vi "S4GUI.vi"(7 "Tab ObsEng":enum32{"Obs", "CCD modes", "Eng"}(tab)) -> ()   [LabVIEW 2018] (continued)
        n4313 = property on="TARGET NAME ASEL" class="Enum (strict)"() -> ("RingText.Text"=w10245:string)  [unwired: 2 in, 2 out]
        n4314 = call "Write target name.vi"("error in (no error)"=w10262, "target name"=w10245, "Optics in"=w10263) -> ("error out"=w10248:errorcluster, "Optics out"=w10249:refnum<class "Opt_Selector.lvclass">)  [unwired: 7 in]
        n4315 = Index Array(array=w10251, index="TARGET NAME ASEL") -> (element=w10250:dbl)
        n4316 = call "Write target.vi"("error in (no error)"=w10248, "target"=w10250, "Optics in"=w10249) -> ("error out"=w10247:errorcluster, "Optics out"=w10246:refnum<class "Opt_Selector.lvclass">)  [unwired: 7 in]
        n4317 = call "Write ASEL.vi"("error in (no error)"=w10247, "Opt_Selector.lvclass"=w10246, "Instrument in"=w10261) -> ("error out"=w10258:errorcluster, "Instrument out"=w10260:refnum<class "Instrument.lvclass">)  [unwired: 7 in]
        n4318 = call "Write Instrument.lvclass.vi"("error in (no error)"=w10258, "Instrument.lvclass"=w10260, "S4ACS_GUI in"=w10259) -> ("error out"=w10255:errorcluster, "S4ACS_GUI out"=w10243:refnum<class "S4GUI.lvclass">)  [unwired: 7 in]
      }
      event "WPROT_stop": Value Change {
        n4319 = event-data() -> ()  [unwired: 1 in, 4 out]
        n4320 = call "Read Instrument.lvclass.vi"("error in (no error)"=w10284, "S4ACS_GUI in"=w10285) -> ("error out"=w10282:errorcluster, "Instrument.lvclass"=w10283:refnum<class "Instrument.lvclass">, "S4ACS_GUI out"=w10269:refnum<class "S4GUI.lvclass">)  [unwired: 7 in]
        n4321 = call "Read WPROT.vi"("error in (no error)"=w10282, "Instrument in"=w10283) -> ("error out"=w10278:errorcluster, "Opt_Selector.lvclass"=w10281:refnum<class "Opt_Selector.lvclass">, "Instrument out"=w10272:refnum<class "Instrument.lvclass">)  [unwired: 7 in]
        n4322 = call-dynamic "Read State Machine.vi"("error in (no error)"=w10278, "Device in"=w10281) -> ("error out"=w10277:errorcluster, "State Machine.lvclass"=w10280:refnum<class "State Machine.lvclass">, "Device out"=w10274:refnum<class "Opt_Selector.lvclass">)  [unwired: 7 in]
        n4323 = call "Next State.vi"("error in (no error)"=w10277, "New_State"=10, "State Machine in"=w10280) -> ("error out"=w10276:errorcluster, "State Machine out"=w10275:refnum<class "State Machine.lvclass">)  [unwired: 7 in]
        n4324 = call-dynamic "Write State Machine.vi"("error in (no error)"=w10276, "State Machine.lvclass"=w10275, "Device in"=w10274) -> ("error out"=w10271:errorcluster, "Device out"=w10273:refnum<class "Opt_Selector.lvclass">)  [unwired: 7 in]
        n4325 = call "Write WPROT.vi"("error in (no error)"=w10271, "Opt_Selector.lvclass"=w10273, "Instrument in"=w10272) -> ("error out"=w10268:errorcluster, "Instrument out"=w10270:refnum<class "Instrument.lvclass">)  [unwired: 7 in]
        n4326 = call "Write Instrument.lvclass.vi"("error in (no error)"=w10268, "Instrument.lvclass"=w10270, "S4ACS_GUI in"=w10269) -> ("error out"=w10267:errorcluster, "S4ACS_GUI out"=w10266:refnum<class "S4GUI.lvclass">)  [unwired: 7 in]
      }
      event "WPROT_init": Value Change {
        n4327 = event-data() -> ()  [unwired: 1 in, 4 out]
        n4328 = call "Read Instrument.lvclass.vi"("error in (no error)"=w10304, "S4ACS_GUI in"=w10305) -> ("error out"=w10302:errorcluster, "Instrument.lvclass"=w10303:refnum<class "Instrument.lvclass">, "S4ACS_GUI out"=w10289:refnum<class "S4GUI.lvclass">)  [unwired: 7 in]
        n4329 = call "Read WPROT.vi"("error in (no error)"=w10302, "Instrument in"=w10303) -> ("error out"=w10298:errorcluster, "Opt_Selector.lvclass"=w10301:refnum<class "Opt_Selector.lvclass">, "Instrument out"=w10292:refnum<class "Instrument.lvclass">)  [unwired: 7 in]
        n4330 = call-dynamic "Read State Machine.vi"("error in (no error)"=w10298, "Device in"=w10301) -> ("error out"=w10297:errorcluster, "State Machine.lvclass"=w10300:refnum<class "State Machine.lvclass">, "Device out"=w10294:refnum<class "Opt_Selector.lvclass">)  [unwired: 7 in]
        n4331 = call "Next State.vi"("error in (no error)"=w10297, "New_State"=30, "State Machine in"=w10300) -> ("error out"=w10296:errorcluster, "State Machine out"=w10295:refnum<class "State Machine.lvclass">)  [unwired: 7 in]
        n4332 = call-dynamic "Write State Machine.vi"("error in (no error)"=w10296, "State Machine.lvclass"=w10295, "Device in"=w10294) -> ("error out"=w10291:errorcluster, "Device out"=w10293:refnum<class "Opt_Selector.lvclass">)  [unwired: 7 in]
        n4333 = call "Write WPROT.vi"("error in (no error)"=w10291, "Opt_Selector.lvclass"=w10293, "Instrument in"=w10292) -> ("error out"=w10288:errorcluster, "Instrument out"=w10290:refnum<class "Instrument.lvclass">)  [unwired: 7 in]
        n4334 = call "Write Instrument.lvclass.vi"("error in (no error)"=w10288, "Instrument.lvclass"=w10290, "S4ACS_GUI in"=w10289) -> ("error out"=w10287:errorcluster, "S4ACS_GUI out"=w10286:refnum<class "S4GUI.lvclass">)  [unwired: 7 in]
      }
      event "WPSEL_target": Value Change {
        n4335 = event-data() -> ("NewVal"=w10315:dbl)  [unwired: 1 in, 3 out]
        n4336 = call "Read Instrument.lvclass.vi"("error in (no error)"=w10319, "S4ACS_GUI in"=w10320) -> ("error out"=w10317:errorcluster, "Instrument.lvclass"=w10318:refnum<class "Instrument.lvclass">, "S4ACS_GUI out"=w10309:refnum<class "S4GUI.lvclass">)  [unwired: 7 in]
        n4337 = call "Read WPSEL.vi"("error in (no error)"=w10317, "Instrument in"=w10318) -> ("error out"=w10314:errorcluster, "Opt_Selector.lvclass"=w10316:refnum<class "Opt_Selector.lvclass">, "Instrument out"=w10312:refnum<class "Instrument.lvclass">)  [unwired: 7 in]
        n4338 = call "Write target.vi"("error in (no error)"=w10314, "target"=w10315, "Optics in"=w10316) -> ("error out"=w10311:errorcluster, "Optics out"=w10313:refnum<class "Opt_Selector.lvclass">)  [unwired: 7 in]
        n4339 = call "Write WPSEL.vi"("error in (no error)"=w10311, "Opt_Selector.lvclass"=w10313, "Instrument in"=w10312) -> ("error out"=w10308:errorcluster, "Instrument out"=w10310:refnum<class "Instrument.lvclass">)  [unwired: 7 in]
        n4340 = call "Write Instrument.lvclass.vi"("error in (no error)"=w10308, "Instrument.lvclass"=w10310, "S4ACS_GUI in"=w10309) -> ("error out"=w10307:errorcluster, "S4ACS_GUI out"=w10306:refnum<class "S4GUI.lvclass">)  [unwired: 7 in]
      }
      event "WPSEL_set": Value Change {
        n4341 = event-data() -> ()  [unwired: 1 in, 4 out]
        n4342 = call "Read Instrument.lvclass.vi"("error in (no error)"=w10339, "S4ACS_GUI in"=w10340) -> ("error out"=w10337:errorcluster, "Instrument.lvclass"=w10338:refnum<class "Instrument.lvclass">, "S4ACS_GUI out"=w10325:refnum<class "S4GUI.lvclass">)  [unwired: 7 in]
        n4343 = call "Read WPSEL.vi"("error in (no error)"=w10337, "Instrument in"=w10338) -> ("error out"=w10334:errorcluster, "Opt_Selector.lvclass"=w10336:refnum<class "Opt_Selector.lvclass">, "Instrument out"=w10328:refnum<class "Instrument.lvclass">)  [unwired: 7 in]
        n4344 = call-dynamic "Read State Machine.vi"("error in (no error)"=w10334, "Device in"=w10336) -> ("error out"=w10333:errorcluster, "State Machine.lvclass"=w10322:refnum<class "State Machine.lvclass">, "Device out"=w10330:refnum<class "Opt_Selector.lvclass">)  [unwired: 7 in]
        n4345 = call "Next State.vi"("error in (no error)"=w10333, "New_State"=1, "State Machine in"=w10322) -> ("error out"=w10332:errorcluster, "State Machine out"=w10331:refnum<class "State Machine.lvclass">)  [unwired: 7 in]
        n4346 = call-dynamic "Write State Machine.vi"("error in (no error)"=w10332, "State Machine.lvclass"=w10331, "Device in"=w10330) -> ("error out"=w10327:errorcluster, "Device out"=w10329:refnum<class "Opt_Selector.lvclass">)  [unwired: 7 in]
        n4347 = call "Write WPSEL.vi"("error in (no error)"=w10327, "Opt_Selector.lvclass"=w10329, "Instrument in"=w10328) -> ("error out"=w10324:errorcluster, "Instrument out"=w10326:refnum<class "Instrument.lvclass">)  [unwired: 7 in]
        n4348 = call "Write Instrument.lvclass.vi"("error in (no error)"=w10324, "Instrument.lvclass"=w10326, "S4ACS_GUI in"=w10325) -> ("error out"=w10323:errorcluster, "S4ACS_GUI out"=w10321:refnum<class "S4GUI.lvclass">)  [unwired: 7 in]
      }
      event "Set Waveplate": Value Change {
        # "OV20230825: Sequência de\nvalores originais."
        # "Garantir que, quando em POLARIMETRIA, pelo menos WP1 esteja selecionado."
        n4349 = event-data() -> ()  [unwired: 1 in, 4 out]
        n4350 = local read "Lambda Selector"() -> (w10444:u16)
        n4351 = property on="Calibrator Selector" class="Ring (strict)"() -> ("RingText.Text"=w10425:string)  [unwired: 2 in, 2 out]
        n4352 = call "Read Instrument.lvclass.vi"("error in (no error)"=w10424, "S4ACS_GUI in"=w10423) -> ("error out"=w10442:errorcluster, "Instrument.lvclass"=w10443:refnum<class "Instrument.lvclass">, "S4ACS_GUI out"=w10440:refnum<class "S4GUI.lvclass">)  [unwired: 7 in]
        n4353 = Build Array(0.0 ("element"), 72.0 ("element"), 144.0 ("element"), 216.0 ("element"), 288.0 ("element")) -> (w10436:dbl[])
        n4354 = local read "Calibrator Selector"() -> (w10426:u16)
        n4355 = Build Array(80.0 ("element"), 0.0 ("element"), 160.0 ("element")) -> (w10470:dbl[])
        n4356 = property on="Lambda Selector" class="Ring (strict)"() -> ("RingText.Text"=w10445:string)  [unwired: 2 in, 2 out]
        n4357 = call "Read CALW.vi"("error in (no error)"=w10442, "Instrument in"=w10443) -> ("error out"=w10434:errorcluster, "Opt_Selector.lvclass"=w10433:refnum<class "Opt_Selector.lvclass">, "Instrument out"=w10441:refnum<class "Instrument.lvclass">)  [unwired: 7 in]
        n4358 = Index Array(array=w10436, index=w10426) -> (element=w10435:dbl)
        n4359 = Index Array(array=w10470, index=w10444) -> (element=w10469:dbl)
        n4360 = case shown="\"OFF\", Default" w10425 {
          tunnel: ["OFF" w10699 "PINHOLE" "SHUTTER" w10704] -> w10343
          frame "OFF", Default {
          }
          frame "POLARIZER" {
            n4361 = disable-structure shown="Enabled" {
              disable-tunnel: ["POLARIZER" "DEPOLARIZER"] -> w10699
              frame Enabled {
              }
              frame Disabled {
                # "OV20230426: Montagem do CALW\nestá com POL e DEPOL invertidos"
              }
            }
          }
          frame "PINHOLE" {
          }
          frame "SHUTTER" {
          }
          frame "DEPOLARIZER" {
            n4362 = disable-structure shown="Enabled" {
              disable-tunnel: ["POLARIZER" "DEPOLARIZER"] -> w10704
              frame Disabled {
                # "OV20230426: Montagem do CALW\nestá com POL e DEPOL invertidos"
              }
              frame Enabled {
              }
            }
          }
        }
        n4363 = call "Write target.vi"("error in (no error)"=w10434, "target"=w10435, "Optics in"=w10433) -> ("error out"=w10431:errorcluster, "Optics out"=w10432:refnum<class "Opt_Selector.lvclass">)  [unwired: 7 in]
        n4364 = case shown="\"OFF\", Default" w10445 {
          tunnel: [w10708 "ON" "ON"] -> w10356
          tunnel: [w10707 w10709 w10712] -> w10461
          tunnel: [w10708 "L/2" "L/4"] -> w10341
          tunnel: [w10707 w10709 w10712] -> w10345
          frame "OFF", Default {
            w10708 = "OFF"
            w10707 = 0.0 ("element")
          }
          frame "Lambda/2" {
            w10709 = 30.0 ("element")
          }
          frame "Lambda/4" {
            w10712 = 30.0 ("element")
          }
        }
        n4365 = call "Write target name.vi"("error in (no error)"=w10431, "target name"=w10343, "Optics in"=w10432) -> ("error out"=w10430:errorcluster, "Optics out"=w10429:refnum<class "Opt_Selector.lvclass">)  [unwired: 7 in]
        n4366 = call "Write CALW.vi"("error in (no error)"=w10430, "Opt_Selector.lvclass"=w10429, "Instrument in"=w10441) -> ("error out"=w10427:errorcluster, "Instrument out"=w10428:refnum<class "Instrument.lvclass">)  [unwired: 7 in]
        n4367 = Equal To 0?(x=w10345) -> (x = 0?=w10346:bool)
        n4368 = call "Write Instrument.lvclass.vi"("error in (no error)"=w10427, "Instrument.lvclass"=w10428, "S4ACS_GUI in"=w10440) -> ("error out"=w10421:errorcluster, "S4ACS_GUI out"=w10422:refnum<class "S4GUI.lvclass">)  [unwired: 7 in]
        n4369 = call "Read Instrument.lvclass.vi"("error in (no error)"=w10421, "S4ACS_GUI in"=w10422) -> ("error out"=w10474:errorcluster, "Instrument.lvclass"=w10454:refnum<class "Instrument.lvclass">, "S4ACS_GUI out"=w10452:refnum<class "S4GUI.lvclass">)  [unwired: 7 in]
        n4370 = call "Read WPSEL.vi"("error in (no error)"=w10474, "Instrument in"=w10454) -> ("error out"=w10460:errorcluster, "Opt_Selector.lvclass"=w10459:refnum<class "Opt_Selector.lvclass">, "Instrument out"=w10453:refnum<class "Instrument.lvclass">)  [unwired: 7 in]
        n4371 = call "Write target.vi"("error in (no error)"=w10460, "target"=w10469, "Optics in"=w10459) -> ("error out"=w10457:errorcluster, "Optics out"=w10458:refnum<class "Opt_Selector.lvclass">)  [unwired: 7 in]
        n4372 = call "Write target name.vi"("error in (no error)"=w10457, "target name"=w10341, "Optics in"=w10458) -> ("error out"=w10456:errorcluster, "Optics out"=w10455:refnum<class "Opt_Selector.lvclass">)  [unwired: 7 in]
        n4373 = call "Write WPSEL.vi"("error in (no error)"=w10456, "Opt_Selector.lvclass"=w10455, "Instrument in"=w10453) -> ("error out"=w10449:errorcluster, "Instrument out"=w10448:refnum<class "Instrument.lvclass">)  [unwired: 7 in]
        n4374 = call "Read ASEL.vi"("error in (no error)"=w10449, "Instrument in"=w10448) -> ("error out"=w10466:errorcluster, "Opt_Selector.lvclass"=w10464:refnum<class "Opt_Selector.lvclass">, "Instrument out"=w10451:refnum<class "Instrument.lvclass">)  [unwired: 7 in]
        n4375 = call "Write target name.vi"("error in (no error)"=w10466, "target name"=w10356, "Optics in"=w10464) -> ("error out"=w10467:errorcluster, "Optics out"=w10463:refnum<class "Opt_Selector.lvclass">)  [unwired: 7 in]
        n4376 = Select(t="OFF", s=w10346, f=w10343) -> (s? t:f=w10344:string)
        n4377 = call "Write target.vi"("error in (no error)"=w10467, "target"=w10461, "Optics in"=w10463) -> ("error out"=w10468:errorcluster, "Optics out"=w10462:refnum<class "Opt_Selector.lvclass">)  [unwired: 7 in]
        n4378 = call "Write ASEL.vi"("error in (no error)"=w10468, "Opt_Selector.lvclass"=w10462, "Instrument in"=w10451) -> ("error out"=w10465:errorcluster, "Instrument out"=w10450:refnum<class "Instrument.lvclass">)  [unwired: 7 in]
        n4379 = call "Write Instrument.lvclass.vi"("error in (no error)"=w10465, "Instrument.lvclass"=w10450, "S4ACS_GUI in"=w10452) -> ("error out"=w10446:errorcluster, "S4ACS_GUI out"=w10447:refnum<class "S4GUI.lvclass">)  [unwired: 7 in]
        n4380 = call "Read Instrument.lvclass.vi"("error in (no error)"=w10446, "S4ACS_GUI in"=w10447) -> ("error out"=w10515:errorcluster, "Instrument.lvclass"=w10516:refnum<class "Instrument.lvclass">, "S4ACS_GUI out"=w10362:refnum<class "S4GUI.lvclass">)  [unwired: 7 in]
        n4381 = call "Read WPSEL.vi"("error in (no error)"=w10515, "Instrument in"=w10516) -> ("error out"=w10512:errorcluster, "Opt_Selector.lvclass"=w10514:refnum<class "Opt_Selector.lvclass">, "Instrument out"=w10506:refnum<class "Instrument.lvclass">)  [unwired: 7 in]
        n4382 = call-dynamic "Read State Machine.vi"("error in (no error)"=w10512, "Device in"=w10514) -> ("error out"=w10511:errorcluster, "State Machine.lvclass"=w10504:refnum<class "State Machine.lvclass">, "Device out"=w10508:refnum<class "Opt_Selector.lvclass">)  [unwired: 7 in]
        n4383 = call "Next State.vi"("error in (no error)"=w10511, "New_State"=1, "State Machine in"=w10504) -> ("error out"=w10510:errorcluster, "State Machine out"=w10509:refnum<class "State Machine.lvclass">)  [unwired: 7 in]
        n4384 = call-dynamic "Write State Machine.vi"("error in (no error)"=w10510, "State Machine.lvclass"=w10509, "Device in"=w10508) -> ("error out"=w10505:errorcluster, "Device out"=w10507:refnum<class "Opt_Selector.lvclass">)  [unwired: 7 in]
        n4385 = call "Write WPSEL.vi"("error in (no error)"=w10505, "Opt_Selector.lvclass"=w10507, "Instrument in"=w10506) -> ("error out"=w10496:errorcluster, "Instrument out"=w10495:refnum<class "Instrument.lvclass">)  [unwired: 7 in]
        n4386 = call "Read ASEL.vi"("error in (no error)"=w10496, "Instrument in"=w10495) -> ("error out"=w10502:errorcluster, "Opt_Selector.lvclass"=w10493:refnum<class "Opt_Selector.lvclass">, "Instrument out"=w10494:refnum<class "Instrument.lvclass">)  [unwired: 7 in]
        n4387 = call-dynamic "Read State Machine.vi"("error in (no error)"=w10502, "Device in"=w10493) -> ("error out"=w10501:errorcluster, "State Machine.lvclass"=w10497:refnum<class "State Machine.lvclass">, "Device out"=w10492:refnum<class "Opt_Selector.lvclass">)  [unwired: 7 in]
        n4388 = call "Next State.vi"("error in (no error)"=w10501, "New_State"=1, "State Machine in"=w10497) -> ("error out"=w10500:errorcluster, "State Machine out"=w10499:refnum<class "State Machine.lvclass">)  [unwired: 7 in]
        n4389 = call-dynamic "Write State Machine.vi"("error in (no error)"=w10500, "State Machine.lvclass"=w10499, "Device in"=w10492) -> ("error out"=w10498:errorcluster, "Device out"=w10491:refnum<class "Opt_Selector.lvclass">)  [unwired: 7 in]
        n4390 = Concatenate Strings("SET WAVEPLATE:  WPSEL=" ("string"), w10341, " CALW=" ("string"), w10344) -> (w10354:string)
        n4391 = call "Write ASEL.vi"("error in (no error)"=w10498, "Opt_Selector.lvclass"=w10491, "Instrument in"=w10494) -> ("error out"=w10478:errorcluster, "Instrument out"=w10480:refnum<class "Instrument.lvclass">)  [unwired: 7 in]
        n4392 = call "Read CALW.vi"("error in (no error)"=w10478, "Instrument in"=w10480) -> ("error out"=w10488:errorcluster, "Opt_Selector.lvclass"=w10490:refnum<class "Opt_Selector.lvclass">, "Instrument out"=w10479:refnum<class "Instrument.lvclass">)  [unwired: 7 in]
        n4393 = call-dynamic "Read State Machine.vi"("error in (no error)"=w10488, "Device in"=w10490) -> ("error out"=w10487:errorcluster, "State Machine.lvclass"=w10481:refnum<class "State Machine.lvclass">, "Device out"=w10484:refnum<class "Opt_Selector.lvclass">)  [unwired: 7 in]
        n4394 = call "Next State.vi"("error in (no error)"=w10487, "New_State"=1, "State Machine in"=w10481) -> ("error out"=w10486:errorcluster, "State Machine out"=w10485:refnum<class "State Machine.lvclass">)  [unwired: 7 in]
        n4395 = call-dynamic "Write State Machine.vi"("error in (no error)"=w10486, "State Machine.lvclass"=w10485, "Device in"=w10484) -> ("error out"=w10482:errorcluster, "Device out"=w10483:refnum<class "Opt_Selector.lvclass">)  [unwired: 7 in]
        n4396 = property on="Lambda Selector" class="Ring (strict)"() -> ("RingText.Text"=w10477:string)  [unwired: 2 in, 2 out]
        n4397 = call "Write CALW.vi"("error in (no error)"=w10482, "Opt_Selector.lvclass"=w10483, "Instrument in"=w10479) -> ("error out"=w10361:errorcluster, "Instrument out"=w10476:refnum<class "Instrument.lvclass">)  [unwired: 7 in]
        n4398 = call-dynamic "Read mode EXPOSE.vi"("error in (no error)"=w10361, "S4GUI in"=w10362) -> ("error out"=w10360:errorcluster, "mode EXPOSE"=w10358:bool, "S4GUI out"=w10359:refnum<class "S4GUI.lvclass">)  [unwired: 7 in]
        n4399 = call-dynamic "Read sync.vi"("error in (no error)"=w10360, "S4ACS_GUI in"=w10359) -> ("error out"=w10378:errorcluster, "sync"=w10377:bool, "S4ACS_GUI out"=w10379:refnum<class "S4GUI.lvclass">)  [unwired: 7 in]
        n4400 = case shown="\"OFF\"" w10477 {
          selector: w10477 -> [w10724 _]
          tunnel: w10476 -> [w10728 w10746]
          tunnel: [w10727 w10746] -> w10475
          tunnel: [w10720 w10745] -> w10395
          tunnel: w10378 -> [w10726 w10745]
          tunnel: [w10717 w10741] -> w10390
          tunnel: w10377 -> [w10716 _]
          tunnel: w10358 -> [w10715 w10744]
          frame "OFF" {
            w10718 = u16 0 items=["OFF", "POLARIZER", "PINHOLE", "SHUTTER", "DEPOLARIZER"] ("Calibrator Selector 2")
            n4401 = call "Read CALW.vi"("error in (no error)"=w10726, "Instrument in"=w10728) -> ("error out"=w10731:errorcluster, "Opt_Selector.lvclass"=w10733:refnum<class "Opt_Selector.lvclass">, "Instrument out"=w10732:refnum<class "Instrument.lvclass">)  [unwired: 7 in]
            n4402 = call "Write target.vi"("error in (no error)"=w10731, "target"=0.0, "Optics in"=w10733) -> ("error out"=w10730:errorcluster, "Optics out"=w10734:refnum<class "Opt_Selector.lvclass">)  [unwired: 7 in]
            n4403 = call "Write target name.vi"("error in (no error)"=w10730, "target name"=w10724, "Optics in"=w10734) -> ("error out"=w10729:errorcluster, "Optics out"=w10735:refnum<class "Opt_Selector.lvclass">)  [unwired: 7 in]
            n4404 = call "Write CALW.vi"("error in (no error)"=w10729, "Opt_Selector.lvclass"=w10735, "Instrument in"=w10732) -> ("error out"=w10719:errorcluster, "Instrument out"=w10727:refnum<class "Instrument.lvclass">)  [unwired: 7 in]
            n4405 = property on="Calibrator Selector" class="Ring (strict)"(error in=w10719, "Value"=w10718, "DisabledEnum"=T12."Disabled and Grayed Out" ("Disabled")) -> (error out=w10721:errorcluster)  [unwired: 1 in, 1 out]
            n4406 = property on="Calibrator Selector" class="Ring (strict)"(error in=w10721, "RingText.Text"="OFF" ("Ring Text.Text")) -> (error out=w10720:errorcluster)  [unwired: 1 in, 1 out]
            n4407 = case shown="True" w10716 {
              tunnel: [u8 0 ("SHUTTER_MODE") w10738] -> w10717
              tunnel: w10715 -> [_ w10737]
              frame False {
                # "Fotom. & Async"
                # "Internal"
              }
              frame True {
                # "Ext. Start"
                # "Internal"
                # "Fotom. Sync. SEM exp mode"
                # "Fotom. Sync. COM exp mode"
                n4408 = Select(t=u8 0, s=w10737, f=u8 6 ("SHUTTER_MODE")) -> (s? t:f=w10738:u8)
              }
            }
          }
          frame Default {
            # "Polar. COM exp mode"
            # "Internal"
            # "Polar. SEM exp mode"
            # "Ext. Start"
            n4409 = Select(t=u8 0, s=w10744, f=u8 6 ("SHUTTER_MODE")) -> (s? t:f=w10741:u8)
          }
        }
        n4410 = call "Write Instrument.lvclass.vi"("error in (no error)"=w10395, "Instrument.lvclass"=w10475, "S4ACS_GUI in"=w10379) -> ("error out"=w10394:errorcluster, "S4ACS_GUI out"=w10383:refnum<class "S4GUI.lvclass">)  [unwired: 7 in]
        n4411 = call-dynamic "Read AcquisitionC.vi"("error in (no error)"=w10394, "S4ACS_GUI in"=w10383) -> ("error out"=w10405:errorcluster, "Acquisition.lvclass"=w10404:refnum<class "Acquisition.lvclass">)  [unwired: 7 in, 1 out]
        n4412 = call-dynamic "Read AcquisitionA.vi"("error in (no error)"=w10394, "S4ACS_GUI in"=w10383) -> ("error out"=w10408:errorcluster, "Acquisition.lvclass"=w10409:refnum<class "Acquisition.lvclass">)  [unwired: 7 in, 1 out]
        n4413 = call "Read AcquisitionB.vi"("error in (no error)"=w10394, "S4ACS_GUI in"=w10383) -> ("error out"=w10406:errorcluster, "Acquisition.lvclass"=w10407:refnum<class "Acquisition.lvclass">)  [unwired: 7 in, 1 out]
        n4414 = call-dynamic "Read AcquisitionD.vi"("error in (no error)"=w10394, "S4ACS_GUI in"=w10383) -> ("error out"=w10402:errorcluster, "Acquisition.lvclass"=w10403:refnum<class "Acquisition.lvclass">)  [unwired: 7 in, 1 out]
        n4415 = call "Read connection.vi"("error in (no error)"=w10405, "Server in"=w10404) -> ("error out"=w10411:errorcluster, "connection"=w10410:bool, "Server out"=w10412:refnum<class "Acquisition.lvclass">)  [unwired: 7 in]
        n4416 = call "Read connection.vi"("error in (no error)"=w10406, "Server in"=w10407) -> ("error out"=w10414:errorcluster, "connection"=w10413:bool, "Server out"=w10415:refnum<class "Acquisition.lvclass">)  [unwired: 7 in]
        n4417 = call "Read connection.vi"("error in (no error)"=w10402, "Server in"=w10403) -> ("error out"=w10391:errorcluster, "connection"=w10392:bool, "Server out"=w10393:refnum<class "Acquisition.lvclass">)  [unwired: 7 in]
        n4418 = call "Read connection.vi"("error in (no error)"=w10408, "Server in"=w10409) -> ("error out"=w10417:errorcluster, "connection"=w10416:bool, "Server out"=w10418:refnum<class "Acquisition.lvclass">)  [unwired: 7 in]
        n4419 = case shown="True" w10410 {
          tunnel: w10412 -> [w10582 w10587]
          tunnel: w10411 -> [w10581 w10586]
          tunnel: [w10582 w10585] -> w10397
          tunnel: [w10581 w10584] -> w10396
          tunnel: w10390 -> [_ w10583]
          frame False {
          }
          frame True {
            # "nome do arquivo .cfg"
            # "seção no arquivo .cfg"
            n4420 = call-dynamic "Read Channel.vi"("error in (no error)"=w10586, "Acquisition in"=w10587) -> ("error out"=w10591:errorcluster, "Channel.lvclass"=w10590:refnum<class "Channel.lvclass">, "Acquisition out"=w10589:refnum<class "Acquisition.lvclass">)  [unwired: 7 in]
            n4421 = call-dynamic "Read Interface.vi"("error in (no error)"=w10591, "Channel in"=w10590) -> ("error out"=w10598:errorcluster, "Interface.lvclass"=w10599:refnum<class "Interface.lvclass">, "Channel out"=w10588:refnum<class "Channel.lvclass">)  [unwired: 7 in]
            n4422 = call-dynamic "Get CCD_Config.vi"("error in (no error)"=w10598, "Interface in"=w10599) -> ("error out"=w10596:errorcluster, "output cluster"=w10595:T30, "Interface out"=w10600:refnum<class "Interface.lvclass">)  [unwired: 7 in]
            n4423 = Bundle By Name(cluster=w10595, "TRIGGER_MODE"=w10583) -> (w10597:T30)
            n4424 = call-dynamic "Set CCD_Config.vi"("error in (no error)"=w10596, "input cluster"=w10597, "Interface in"=w10600) -> ("error out"=w10594:errorcluster, "Interface out"=w10601:refnum<class "Interface.lvclass">)  [unwired: 7 in]
            n4425 = Flatten To String(anything=w10597, error in (no error)=w10594) -> (data string=w10592:string, error out=w10593:errorcluster)  [unwired: 2 in, 1 out]
            n4426 = call "Write flatted cluster.vi"("error in (no error)"=w10593, "flatted cluster"=w10592, "Interface in"=w10601) -> ("error out"=w10603:errorcluster, "Interface out"=w10602:refnum<class "Interface.lvclass">)  [unwired: 7 in]
            n4427 = call-dynamic "Write Interface.vi"("error in (no error)"=w10603, "Interface.lvclass"=w10602, "Channel in"=w10588) -> ("error out"=w10609:errorcluster, "Channel out"=w10610:refnum<class "Channel.lvclass">)  [unwired: 7 in]
            n4428 = call "Write section_name.vi"("error in (no error)"=w10609, "section_name"="CCD_ACS3", "Channel in"=w10610) -> ("error out"=w10607:errorcluster, "Channel out"=w10613:refnum<class "Channel.lvclass">)  [unwired: 7 in]
            n4429 = call-dynamic "save config.vi"("error in (no error)"=w10607, "file config"="lastsaved.cfg", "Channel in"=w10613) -> ("error out"=w10608:errorcluster, "Channel out"=w10614:refnum<class "Channel.lvclass">)  [unwired: 7 in]
            n4430 = call-dynamic "Read State Machine.vi"("error in (no error)"=w10608, "Device in"=w10614) -> ("error out"=w10604:errorcluster, "State Machine.lvclass"=w10616:refnum<class "State Machine.lvclass">, "Device out"=w10615:refnum<class "Channel.lvclass">)  [unwired: 7 in]
            n4431 = call-dynamic "Write State.vi"("error in (no error)"=w10604, "State"=60, "State Machine in"=w10616) -> ("error out"=w10605:errorcluster, "State Machine out"=w10617:refnum<class "State Machine.lvclass">)  [unwired: 7 in]
            n4432 = call-dynamic "Write State Machine.vi"("error in (no error)"=w10605, "State Machine.lvclass"=w10617, "Device in"=w10615) -> ("error out"=w10619:errorcluster, "Device out"=w10618:refnum<class "Channel.lvclass">)  [unwired: 7 in]
            n4433 = call-dynamic "Write Channel.vi"("error in (no error)"=w10619, "Channel.lvclass"=w10618, "Acquisition in"=w10589) -> ("error out"=w10584:errorcluster, "Acquisition out"=w10585:refnum<class "Acquisition.lvclass">)  [unwired: 7 in]
          }
        }
        n4434 = case shown="True" w10392 {
          tunnel: w10393 -> [w10543 w10548]
          tunnel: w10391 -> [w10542 w10547]
          tunnel: w10390 -> [_ w10546]
          tunnel: [w10543 w10545] -> w10389
          tunnel: [w10542 w10544] -> w10388
          frame False {
          }
          frame True {
            # "nome do arquivo .cfg"
            # "seção no arquivo .cfg"
            n4435 = call-dynamic "Read Channel.vi"("error in (no error)"=w10547, "Acquisition in"=w10548) -> ("error out"=w10577:errorcluster, "Channel.lvclass"=w10578:refnum<class "Channel.lvclass">, "Acquisition out"=w10579:refnum<class "Acquisition.lvclass">)  [unwired: 7 in]
            n4436 = call-dynamic "Read Interface.vi"("error in (no error)"=w10577, "Channel in"=w10578) -> ("error out"=w10570:errorcluster, "Interface.lvclass"=w10569:refnum<class "Interface.lvclass">, "Channel out"=w10580:refnum<class "Channel.lvclass">)  [unwired: 7 in]
            n4437 = call-dynamic "Get CCD_Config.vi"("error in (no error)"=w10570, "Interface in"=w10569) -> ("error out"=w10572:errorcluster, "output cluster"=w10573:T30, "Interface out"=w10568:refnum<class "Interface.lvclass">)  [unwired: 7 in]
            n4438 = Bundle By Name(cluster=w10573, "TRIGGER_MODE"=w10546) -> (w10571:T30)
            n4439 = call-dynamic "Set CCD_Config.vi"("error in (no error)"=w10572, "input cluster"=w10571, "Interface in"=w10568) -> ("error out"=w10574:errorcluster, "Interface out"=w10567:refnum<class "Interface.lvclass">)  [unwired: 7 in]
            n4440 = Flatten To String(anything=w10571, error in (no error)=w10574) -> (data string=w10576:string, error out=w10575:errorcluster)  [unwired: 2 in, 1 out]
            n4441 = call "Write flatted cluster.vi"("error in (no error)"=w10575, "flatted cluster"=w10576, "Interface in"=w10567) -> ("error out"=w10565:errorcluster, "Interface out"=w10566:refnum<class "Interface.lvclass">)  [unwired: 7 in]
            n4442 = call-dynamic "Write Interface.vi"("error in (no error)"=w10565, "Interface.lvclass"=w10566, "Channel in"=w10580) -> ("error out"=w10559:errorcluster, "Channel out"=w10558:refnum<class "Channel.lvclass">)  [unwired: 7 in]
            n4443 = call "Write section_name.vi"("error in (no error)"=w10559, "section_name"="CCD_ACS4", "Channel in"=w10558) -> ("error out"=w10561:errorcluster, "Channel out"=w10555:refnum<class "Channel.lvclass">)  [unwired: 7 in]
            n4444 = call-dynamic "save config.vi"("error in (no error)"=w10561, "file config"="lastsaved.cfg", "Channel in"=w10555) -> ("error out"=w10560:errorcluster, "Channel out"=w10554:refnum<class "Channel.lvclass">)  [unwired: 7 in]
            n4445 = call-dynamic "Read State Machine.vi"("error in (no error)"=w10560, "Device in"=w10554) -> ("error out"=w10564:errorcluster, "State Machine.lvclass"=w10552:refnum<class "State Machine.lvclass">, "Device out"=w10553:refnum<class "Channel.lvclass">)  [unwired: 7 in]
            n4446 = call-dynamic "Write State.vi"("error in (no error)"=w10564, "State"=60, "State Machine in"=w10552) -> ("error out"=w10563:errorcluster, "State Machine out"=w10551:refnum<class "State Machine.lvclass">)  [unwired: 7 in]
            n4447 = call-dynamic "Write State Machine.vi"("error in (no error)"=w10563, "State Machine.lvclass"=w10551, "Device in"=w10553) -> ("error out"=w10549:errorcluster, "Device out"=w10550:refnum<class "Channel.lvclass">)  [unwired: 7 in]
            n4448 = call-dynamic "Write Channel.vi"("error in (no error)"=w10549, "Channel.lvclass"=w10550, "Acquisition in"=w10579) -> ("error out"=w10544:errorcluster, "Acquisition out"=w10545:refnum<class "Acquisition.lvclass">)  [unwired: 7 in]
          }
        }
        n4449 = case shown="True" w10413 {
          tunnel: w10415 -> [w10621 w10626]
          tunnel: w10414 -> [w10620 w10625]
          tunnel: [w10621 w10624] -> w10399
          tunnel: [w10620 w10623] -> w10398
          tunnel: w10390 -> [_ w10622]
          frame False {
          }
          frame True {
            # "nome do arquivo .cfg"
            # "seção no arquivo .cfg"
            n4450 = call-dynamic "Read Channel.vi"("error in (no error)"=w10625, "Acquisition in"=w10626) -> ("error out"=w10630:errorcluster, "Channel.lvclass"=w10629:refnum<class "Channel.lvclass">, "Acquisition out"=w10628:refnum<class "Acquisition.lvclass">)  [unwired: 7 in]
            n4451 = call-dynamic "Read Interface.vi"("error in (no error)"=w10630, "Channel in"=w10629) -> ("error out"=w10637:errorcluster, "Interface.lvclass"=w10638:refnum<class "Interface.lvclass">, "Channel out"=w10627:refnum<class "Channel.lvclass">)  [unwired: 7 in]
            n4452 = call-dynamic "Get CCD_Config.vi"("error in (no error)"=w10637, "Interface in"=w10638) -> ("error out"=w10635:errorcluster, "output cluster"=w10634:T30, "Interface out"=w10639:refnum<class "Interface.lvclass">)  [unwired: 7 in]
            n4453 = Bundle By Name(cluster=w10634, "TRIGGER_MODE"=w10622) -> (w10636:T30)
            n4454 = call-dynamic "Set CCD_Config.vi"("error in (no error)"=w10635, "input cluster"=w10636, "Interface in"=w10639) -> ("error out"=w10633:errorcluster, "Interface out"=w10640:refnum<class "Interface.lvclass">)  [unwired: 7 in]
            n4455 = Flatten To String(anything=w10636, error in (no error)=w10633) -> (data string=w10631:string, error out=w10632:errorcluster)  [unwired: 2 in, 1 out]
            n4456 = call "Write flatted cluster.vi"("error in (no error)"=w10632, "flatted cluster"=w10631, "Interface in"=w10640) -> ("error out"=w10642:errorcluster, "Interface out"=w10641:refnum<class "Interface.lvclass">)  [unwired: 7 in]
            n4457 = call-dynamic "Write Interface.vi"("error in (no error)"=w10642, "Interface.lvclass"=w10641, "Channel in"=w10627) -> ("error out"=w10648:errorcluster, "Channel out"=w10649:refnum<class "Channel.lvclass">)  [unwired: 7 in]
            n4458 = call "Write section_name.vi"("error in (no error)"=w10648, "section_name"="CCD_ACS2", "Channel in"=w10649) -> ("error out"=w10646:errorcluster, "Channel out"=w10652:refnum<class "Channel.lvclass">)  [unwired: 7 in]
            n4459 = call-dynamic "save config.vi"("error in (no error)"=w10646, "file config"="lastsaved.cfg", "Channel in"=w10652) -> ("error out"=w10647:errorcluster, "Channel out"=w10653:refnum<class "Channel.lvclass">)  [unwired: 7 in]
            n4460 = call-dynamic "Read State Machine.vi"("error in (no error)"=w10647, "Device in"=w10653) -> ("error out"=w10643:errorcluster, "State Machine.lvclass"=w10655:refnum<class "State Machine.lvclass">, "Device out"=w10654:refnum<class "Channel.lvclass">)  [unwired: 7 in]
            n4461 = call-dynamic "Write State.vi"("error in (no error)"=w10643, "State"=60, "State Machine in"=w10655) -> ("error out"=w10644:errorcluster, "State Machine out"=w10656:refnum<class "State Machine.lvclass">)  [unwired: 7 in]
            n4462 = call-dynamic "Write State Machine.vi"("error in (no error)"=w10644, "State Machine.lvclass"=w10656, "Device in"=w10654) -> ("error out"=w10658:errorcluster, "Device out"=w10657:refnum<class "Channel.lvclass">)  [unwired: 7 in]
            n4463 = call-dynamic "Write Channel.vi"("error in (no error)"=w10658, "Channel.lvclass"=w10657, "Acquisition in"=w10628) -> ("error out"=w10623:errorcluster, "Acquisition out"=w10624:refnum<class "Acquisition.lvclass">)  [unwired: 7 in]
          }
        }
        n4464 = case shown="True" w10416 {
          tunnel: [w10659 w10693] -> w10400
          tunnel: [w10660 w10692] -> w10401
          tunnel: w10418 -> [w10660 w10663]
          tunnel: w10417 -> [w10659 w10662]
          tunnel: w10390 -> [_ w10661]
          frame False {
          }
          frame True {
            # "nome do arquivo .cfg"
            # "seção no arquivo .cfg"
            n4465 = call-dynamic "Read Channel.vi"("error in (no error)"=w10662, "Acquisition in"=w10663) -> ("error out"=w10694:errorcluster, "Channel.lvclass"=w10695:refnum<class "Channel.lvclass">, "Acquisition out"=w10696:refnum<class "Acquisition.lvclass">)  [unwired: 7 in]
            n4466 = call-dynamic "Read Interface.vi"("error in (no error)"=w10694, "Channel in"=w10695) -> ("error out"=w10685:errorcluster, "Interface.lvclass"=w10684:refnum<class "Interface.lvclass">, "Channel out"=w10697:refnum<class "Channel.lvclass">)  [unwired: 7 in]
            n4467 = call-dynamic "Get CCD_Config.vi"("error in (no error)"=w10685, "Interface in"=w10684) -> ("error out"=w10687:errorcluster, "output cluster"=w10688:T30, "Interface out"=w10683:refnum<class "Interface.lvclass">)  [unwired: 7 in]
            n4468 = Bundle By Name(cluster=w10688, "TRIGGER_MODE"=w10661) -> (w10686:T30)
            n4469 = call-dynamic "Set CCD_Config.vi"("error in (no error)"=w10687, "input cluster"=w10686, "Interface in"=w10683) -> ("error out"=w10689:errorcluster, "Interface out"=w10682:refnum<class "Interface.lvclass">)  [unwired: 7 in]
            n4470 = Flatten To String(anything=w10686, error in (no error)=w10689) -> (data string=w10691:string, error out=w10690:errorcluster)  [unwired: 2 in, 1 out]
            n4471 = call "Write flatted cluster.vi"("error in (no error)"=w10690, "flatted cluster"=w10691, "Interface in"=w10682) -> ("error out"=w10680:errorcluster, "Interface out"=w10681:refnum<class "Interface.lvclass">)  [unwired: 7 in]
            n4472 = call-dynamic "Write Interface.vi"("error in (no error)"=w10680, "Interface.lvclass"=w10681, "Channel in"=w10697) -> ("error out"=w10675:errorcluster, "Channel out"=w10674:refnum<class "Channel.lvclass">)  [unwired: 7 in]
            n4473 = call "Write section_name.vi"("error in (no error)"=w10675, "section_name"="CCD_ACS1", "Channel in"=w10674) -> ("error out"=w10676:errorcluster, "Channel out"=w10671:refnum<class "Channel.lvclass">)  [unwired: 7 in]
            n4474 = call-dynamic "save config.vi"("error in (no error)"=w10676, "file config"="lastsaved.cfg", "Channel in"=w10671) -> ("error out"=w10664:errorcluster, "Channel out"=w10665:refnum<class "Channel.lvclass">)  [unwired: 7 in]
            n4475 = call-dynamic "Read State Machine.vi"("error in (no error)"=w10664, "Device in"=w10665) -> ("error out"=w10679:errorcluster, "State Machine.lvclass"=w10669:refnum<class "State Machine.lvclass">, "Device out"=w10670:refnum<class "Channel.lvclass">)  [unwired: 7 in]
            n4476 = call-dynamic "Write State.vi"("error in (no error)"=w10679, "State"=60, "State Machine in"=w10669) -> ("error out"=w10678:errorcluster, "State Machine out"=w10668:refnum<class "State Machine.lvclass">)  [unwired: 7 in]
            n4477 = call-dynamic "Write State Machine.vi"("error in (no error)"=w10678, "State Machine.lvclass"=w10668, "Device in"=w10670) -> ("error out"=w10666:errorcluster, "Device out"=w10667:refnum<class "Channel.lvclass">)  [unwired: 7 in]
            n4478 = call-dynamic "Write Channel.vi"("error in (no error)"=w10666, "Channel.lvclass"=w10667, "Acquisition in"=w10696) -> ("error out"=w10693:errorcluster, "Acquisition out"=w10692:refnum<class "Acquisition.lvclass">)  [unwired: 7 in]
          }
        }
        n4479 = call-dynamic "Write AcquisitionA.vi"("error in (no error)"=w10400, "Acquisition.lvclass"=w10401, "S4ACS_GUI in"=w10383) -> ("error out"=w10387:errorcluster, "S4ACS_GUI out"=w10382:refnum<class "S4GUI.lvclass">)  [unwired: 7 in]
        n4480 = call "Write AcquisitionB.vi"("error in (no error)"=w10398, "Acquisition.lvclass"=w10399, "S4ACS_GUI in"=w10382) -> ("error out"=w10386:errorcluster, "S4ACS_GUI out"=w10381:refnum<class "S4GUI.lvclass">)  [unwired: 7 in]
        n4481 = call-dynamic "Write AcquisitionC.vi"("error in (no error)"=w10396, "Acquisition.lvclass"=w10397, "S4ACS_GUI in"=w10381) -> ("error out"=w10385:errorcluster, "S4ACS_GUI out"=w10380:refnum<class "S4GUI.lvclass">)  [unwired: 7 in]
        n4482 = call-dynamic "Write AcquisitionD.vi"("error in (no error)"=w10388, "Acquisition.lvclass"=w10389, "S4ACS_GUI in"=w10380) -> ("error out"=w10384:errorcluster, "S4ACS_GUI out"=w10364:refnum<class "S4GUI.lvclass">)  [unwired: 7 in]
        n4483 = Merge Errors(w10387, w10386, w10385, w10384) -> (w10363:errorcluster)
        n4484 = call "Read Instrument.lvclass.vi"("error in (no error)"=w10363, "S4ACS_GUI in"=w10364) -> ("error out"=w10369:errorcluster, "Instrument.lvclass"=w10368:refnum<class "Instrument.lvclass">, "S4ACS_GUI out"=w10365:refnum<class "S4GUI.lvclass">)  [unwired: 7 in]
        n4485 = call "Read ASEL.vi"("error in (no error)"=w10369, "Instrument in"=w10368) -> ("error out"=w10376:errorcluster, "Opt_Selector.lvclass"=w10375:refnum<class "Opt_Selector.lvclass">, "Instrument out"=w10374:refnum<class "Instrument.lvclass">)  [unwired: 7 in]
        n4486 = call "Read target name.vi"("error in (no error)"=w10376, "Optics in"=w10375) -> ("error out"=w10372:errorcluster, "target name"=w10352:string, "Optics out"=w10373:refnum<class "Opt_Selector.lvclass">)  [unwired: 7 in]
        n4487 = call "Write ASEL.vi"("error in (no error)"=w10372, "Opt_Selector.lvclass"=w10373, "Instrument in"=w10374) -> ("error out"=w10371:errorcluster, "Instrument out"=w10367:refnum<class "Instrument.lvclass">)  [unwired: 7 in]
        n4488 = Concatenate Strings(w10354, " ASEL=" ("string"), w10352) -> (w10349:string)
        n4489 = case shown="\"ON\"" w10352 {
          tunnel: w10371 -> [w10518 w10529]
          tunnel: [w10518 w10525] -> w10370
          tunnel: w10367 -> [w10517 w10530]
          tunnel: [w10517 w10526] -> w10366
          frame Default {
          }
          frame "ON" {
            n4490 = call "Read WPROT.vi"("error in (no error)"=w10529, "Instrument in"=w10530) -> ("error out"=w10521:errorcluster, "Opt_Selector.lvclass"=w10528:refnum<class "Opt_Selector.lvclass">, "Instrument out"=w10527:refnum<class "Instrument.lvclass">)  [unwired: 7 in]
            n4491 = call-dynamic "Read sequencia.vi"("error in (no error)"=w10521, "Opt_Selector in"=w10528) -> ("error out"=w10520:errorcluster, "sequencia"=w10524:u16, "Opt_Selector out"=w10523:refnum<class "Opt_Selector.lvclass">)  [unwired: 7 in]
            n4492 = case shown="0" w10524 {
              tunnel: w10523 -> [w10532 w10541]
              tunnel: [w10532 w10537] -> w10522
              tunnel: w10520 -> [w10531 w10540]
              tunnel: [w10531 w10535] -> w10519
              frame Default {
              }
              frame 0 {
                n4493 = call-dynamic "Write sequencia.vi"("error in (no error)"=w10540, "sequencia"=u16 1, "Opt_Selector in"=w10541) -> ("error out"=w10536:errorcluster, "Opt_Selector out"=w10538:refnum<class "Opt_Selector.lvclass">)  [unwired: 7 in]
                n4494 = local write "P0"(TRUE ("P0")) -> ()
                n4495 = call-dynamic "Write sequencia_ant.vi"("error in (no error)"=w10536, "sequencia_ant"=u16 1, "Opt_Selector in"=w10538) -> ("error out"=w10535:errorcluster, "Opt_Selector out"=w10537:refnum<class "Opt_Selector.lvclass">)  [unwired: 7 in]
              }
            }
            n4496 = call "Write WPROT.vi"("error in (no error)"=w10519, "Opt_Selector.lvclass"=w10522, "Instrument in"=w10527) -> ("error out"=w10525:errorcluster, "Instrument out"=w10526:refnum<class "Instrument.lvclass">)  [unwired: 7 in]
          }
        }
        n4497 = call "Write Instrument.lvclass.vi"("error in (no error)"=w10370, "Instrument.lvclass"=w10366, "S4ACS_GUI in"=w10365) -> ("error out"=w10350:errorcluster, "S4ACS_GUI out"=w10351:refnum<class "S4GUI.lvclass">)  [unwired: 7 in]
        n4498 = call-dynamic "Write User Event.vi"("error in (no error)"=w10350, "User Event"=w10349, "S4GUI in"=w10351) -> ("error out"=w10347:errorcluster, "S4GUI out"=w10348:refnum<class "S4GUI.lvclass">)  [unwired: 7 in]
      }
      event "Init mode": Value Change {
        n4499 = event-data() -> ()  [unwired: 1 in, 4 out]
        n4500 = call-dynamic "Write User Event.vi"("error in (no error)"=w10750, "User Event"="INIT INSTRUMENT CLICKED", "S4GUI in"=w10751) -> ("error out"=w10748:errorcluster, "S4GUI out"=w10749:refnum<class "S4GUI.lvclass">)  [unwired: 7 in]
        n4501 = call-dynamic "Read Obs_state.vi"("error in (no error)"=w10748, "S4ACS_GUI in"=w10749) -> ("error out"=w10752:errorcluster, "Obs_state"=w10754:u32, "S4ACS_GUI out"=w10755:refnum<class "S4GUI.lvclass">)  [unwired: 7 in]
        n4502 = In Range and Coerce(upper limit=u32 226, x=w10754, lower limit=u32 220 ("upper limit")) -> (In Range?=w10753:bool)  [unwired: 1 out]
        n4503 = case shown="False" w10753 {
          tunnel: [w10763 w10771] -> w10759
          tunnel: [w10762 w10769] -> w10758
          tunnel: w10752 -> [w10761 w10770]
          tunnel: w10755 -> [w10760 w10772]
          frame False {
            n4504 = call-dynamic "Write sync.vi"("error in (no error)"=w10761, "sync"=TRUE, "S4ACS_GUI in"=w10760) -> ("error out"=w10765:errorcluster, "S4ACS_GUI out"=w10764:refnum<class "S4GUI.lvclass">)  [unwired: 7 in]
            n4505 = call-dynamic "Write Obs_state.vi"("error in (no error)"=w10765, "Obs_state"=u32 220, "S4ACS_GUI in"=w10764) -> ("error out"=w10762:errorcluster, "S4ACS_GUI out"=w10763:refnum<class "S4GUI.lvclass">)  [unwired: 7 in]
          }
          frame True {
            n4506 = call-dynamic "Write Obs_state.vi"("error in (no error)"=w10770, "Obs_state"=u32 0, "S4ACS_GUI in"=w10772) -> ("error out"=w10769:errorcluster, "S4ACS_GUI out"=w10771:refnum<class "S4GUI.lvclass">)  [unwired: 7 in]
          }
        }
      }
      event "exit": Value Change {
        # "Se Instrument.lvclass estiver operacional, faz o parking.\nCaso contrário, encerra imediatamente."
        n4507 = event-data() -> ()  [unwired: 1 in, 4 out]
        n4508 = call-dynamic "Write User Event.vi"("error in (no error)"=w10781, "User Event"="EXIT APP CLICKED", "S4GUI in"=w10782) -> ("error out"=w10776:errorcluster, "S4GUI out"=w10777:refnum<class "S4GUI.lvclass">)  [unwired: 7 in]
        n4509 = call "Read Instrument.lvclass.vi"("error in (no error)"=w10776, "S4ACS_GUI in"=w10777) -> ("error out"=w10773:errorcluster, "Instrument.lvclass"=w10775:refnum<class "Instrument.lvclass">, "S4ACS_GUI out"=w10779:refnum<class "S4GUI.lvclass">)  [unwired: 7 in]
        n4510 = call-dynamic "Read operational.vi"("error in (no error)"=w10773, "Server in"=w10775) -> ("error out"=w10778:errorcluster, "operational"=w10774:bool)  [unwired: 7 in, 1 out]
        n4511 = case shown="True" w10774 {
          tunnel: [w10786 w10799] -> w10784
          tunnel: [w10785 w10798] -> w10783
          tunnel: w10779 -> [w10789 w10790]
          tunnel: w10778 -> [w10788 w10791]
          frame False {
            n4512 = call-dynamic "Write exit.vi"("error in (no error)"=w10788, "exit"=TRUE, "S4GUI in"=w10789) -> ("error out"=w10785:errorcluster, "S4GUI out"=w10786:refnum<class "S4GUI.lvclass">)  [unwired: 7 in]
          }
          frame True {
            n4513 = call-dynamic "Read Obs_state.vi"("error in (no error)"=w10791, "S4ACS_GUI in"=w10790) -> ("error out"=w10792:errorcluster, "Obs_state"=w10794:u32, "S4ACS_GUI out"=w10795:refnum<class "S4GUI.lvclass">)  [unwired: 7 in]
            n4514 = In Range and Coerce(upper limit=u32 234, x=w10794, lower limit=u32 230 ("upper limit")) -> (In Range?=w10793:bool)  [unwired: 1 out]
            n4515 = case shown="False" w10793 {
              tunnel: [w10805 w10822] -> w10799
              tunnel: [w10804 w10821] -> w10798
              tunnel: w10792 -> [w10807 w10821]
              tunnel: w10795 -> [w10806 w10822]
              frame False {
                n4516 = Two Button Dialog(message="Park before exiting?", 1:"NO" ("F button name (\"Cancel\")"), 2:"YES" ("T button name (\"OK\")")) -> (T button?=w10800:bool)
                n4517 = case shown="True" w10800 {
                  tunnel: w10807 -> [w10811 w10816]
                  tunnel: w10806 -> [w10810 w10815]
                  tunnel: [w10809 w10814] -> w10805
                  tunnel: [w10808 w10813] -> w10804
                  frame False {
                    n4518 = call-dynamic "Write exit.vi"("error in (no error)"=w10811, "exit"=TRUE, "S4GUI in"=w10810) -> ("error out"=w10808:errorcluster, "S4GUI out"=w10809:refnum<class "S4GUI.lvclass">)  [unwired: 7 in]
                  }
                  frame True {
                    n4519 = call-dynamic "Write sync.vi"("error in (no error)"=w10816, "sync"=TRUE, "S4ACS_GUI in"=w10815) -> ("error out"=w10818:errorcluster, "S4ACS_GUI out"=w10817:refnum<class "S4GUI.lvclass">)  [unwired: 7 in]
                    n4520 = call-dynamic "Write Obs_state.vi"("error in (no error)"=w10818, "Obs_state"=u32 230, "S4ACS_GUI in"=w10817) -> ("error out"=w10813:errorcluster, "S4ACS_GUI out"=w10814:refnum<class "S4GUI.lvclass">)  [unwired: 7 in]
                  }
                }
              }
              frame True {
              }
            }
          }
        }
      }
      event "WPSEL_stop": Value Change {
        n4521 = event-data() -> ()  [unwired: 1 in, 4 out]
        n4522 = call "Read Instrument.lvclass.vi"("error in (no error)"=w10841, "S4ACS_GUI in"=w10842) -> ("error out"=w10839:errorcluster, "Instrument.lvclass"=w10840:refnum<class "Instrument.lvclass">, "S4ACS_GUI out"=w10826:refnum<class "S4GUI.lvclass">)  [unwired: 7 in]
        n4523 = call "Read WPSEL.vi"("error in (no error)"=w10839, "Instrument in"=w10840) -> ("error out"=w10835:errorcluster, "Opt_Selector.lvclass"=w10838:refnum<class "Opt_Selector.lvclass">, "Instrument out"=w10829:refnum<class "Instrument.lvclass">)  [unwired: 7 in]
        n4524 = call-dynamic "Read State Machine.vi"("error in (no error)"=w10835, "Device in"=w10838) -> ("error out"=w10834:errorcluster, "State Machine.lvclass"=w10837:refnum<class "State Machine.lvclass">, "Device out"=w10831:refnum<class "Opt_Selector.lvclass">)  [unwired: 7 in]
        n4525 = call "Next State.vi"("error in (no error)"=w10834, "New_State"=10, "State Machine in"=w10837) -> ("error out"=w10833:errorcluster, "State Machine out"=w10832:refnum<class "State Machine.lvclass">)  [unwired: 7 in]
        n4526 = call-dynamic "Write State Machine.vi"("error in (no error)"=w10833, "State Machine.lvclass"=w10832, "Device in"=w10831) -> ("error out"=w10828:errorcluster, "Device out"=w10830:refnum<class "Opt_Selector.lvclass">)  [unwired: 7 in]
        n4527 = call "Write WPSEL.vi"("error in (no error)"=w10828, "Opt_Selector.lvclass"=w10830, "Instrument in"=w10829) -> ("error out"=w10825:errorcluster, "Instrument out"=w10827:refnum<class "Instrument.lvclass">)  [unwired: 7 in]
        n4528 = call "Write Instrument.lvclass.vi"("error in (no error)"=w10825, "Instrument.lvclass"=w10827, "S4ACS_GUI in"=w10826) -> ("error out"=w10824:errorcluster, "S4ACS_GUI out"=w10823:refnum<class "S4GUI.lvclass">)  [unwired: 7 in]
      }
      event "WPSEL_init": Value Change {
        n4529 = event-data() -> ()  [unwired: 1 in, 4 out]
        n4530 = call "Read Instrument.lvclass.vi"("error in (no error)"=w10861, "S4ACS_GUI in"=w10862) -> ("error out"=w10859:errorcluster, "Instrument.lvclass"=w10860:refnum<class "Instrument.lvclass">, "S4ACS_GUI out"=w10846:refnum<class "S4GUI.lvclass">)  [unwired: 7 in]
        n4531 = call "Read WPSEL.vi"("error in (no error)"=w10859, "Instrument in"=w10860) -> ("error out"=w10855:errorcluster, "Opt_Selector.lvclass"=w10858:refnum<class "Opt_Selector.lvclass">, "Instrument out"=w10849:refnum<class "Instrument.lvclass">)  [unwired: 7 in]
        n4532 = call-dynamic "Read State Machine.vi"("error in (no error)"=w10855, "Device in"=w10858) -> ("error out"=w10854:errorcluster, "State Machine.lvclass"=w10857:refnum<class "State Machine.lvclass">, "Device out"=w10851:refnum<class "Opt_Selector.lvclass">)  [unwired: 7 in]
        n4533 = call "Next State.vi"("error in (no error)"=w10854, "New_State"=30, "State Machine in"=w10857) -> ("error out"=w10853:errorcluster, "State Machine out"=w10852:refnum<class "State Machine.lvclass">)  [unwired: 7 in]
        n4534 = call-dynamic "Write State Machine.vi"("error in (no error)"=w10853, "State Machine.lvclass"=w10852, "Device in"=w10851) -> ("error out"=w10848:errorcluster, "Device out"=w10850:refnum<class "Opt_Selector.lvclass">)  [unwired: 7 in]
